vi "Read Firmware Version.vi"(8 "Error In":errorcluster, 11 "ChipKit Resource in":T1={"COM Port"="", "Board Type"=enum."ChipKit Uno32", "Connection Type"=enum."USB / Serial", "Baud Rate (115200)"=15, "Bytes Per Packet (15)"=15}) -> (0 "Error Out":errorcluster, 3 "ChipKit Resource out":T1={"COM Port"="", "Board Type"=enum."ChipKit Uno32", "Connection Type"=enum."USB / Serial", "Baud Rate (115200)"=15, "Bytes Per Packet (15)"=15})   [LabVIEW 2011, in "LabVIEW Interface for ChipKit.lvlib"]
uses:
  LabVIEW Interface for ChipKit.lvlib
  Private/Type Defs/Command.ctl
  Private/Type Defs/Board Type.ctl
  Private/Type Defs/Connection Type.ctl
  Private/Type Defs/Chipkit Resource.ctl
panel:
  out "Firmware Version":string
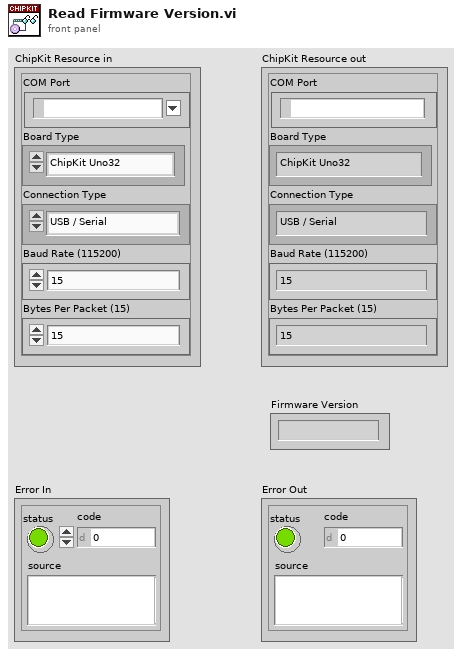
[diagram p1: front panel]
types:
  T1 = typedef "LabVIEW Interface for ChipKit.lvlib/Chipkit Resource.ctl" = cluster{"COM Port":refnum<visa-resource-name>, "Board Type":T2, "Connection Type":T3, "Baud Rate (115200)":u32, "Bytes Per Packet (15)":u32}
  T2 = typedef "LabVIEW Interface for ChipKit.lvlib/Board Type.ctl" = enum16{"ChipKit uC32", "ChipKit Uno32", "ChipKit Max32"}
  T3 = typedef "LabVIEW Interface for ChipKit.lvlib/Connection Type.ctl" = enum8{"USB / Serial", "XBEE", "BlueSmirf (Bluetooth)"}
  T4 = typedef "LabVIEW Interface for ChipKit.lvlib/Command.ctl" = enum8{"setArduinoMode", "flushSerial", "setPinMode", "digitalWritePin", "digitalWritePort", "tone", "digitalReadPin", "digitalReadPort", "analogReadPin", "analogReadPort", "pwmWritePin", "pwmWritePort", "sevenSegment_Configure", "sevenSegment_Write", "I2C Init", "I2C Write", "I2C Read", "SPI Init", "SPI Set Bit Order", "SPI Set Clock Divider", "SPI Set Data Mode", "SPI Send / Receive", "SPI Close", "Servo Set Num Servos", "Servo Config Servo", "Servo Write Angle", "Servo Read Angle", "Servo Write Pulse Width", "Servo Read Pulse Width", "Servo Detach", "LCD Init", "LCD Set Size", "LCD Set Cursor Mode", "LCD Clear", "LCD Set Cursor Position", "LCD Print", "LCD Display Power", "LCD Scroll Display", "LCD Autoscroll", "LCD Print Direction", "LCD Create Custom Char", "LCD Print Custom Char", "contAcqOn", "contAcqOff", "getFirmwareVersion", "FiniteSampleStart", "NA", "NA2", "Conifg Stepper", "Stepper Write", "Stepper Detach", "Stepper Steps To Go", "Config DO Port", "Config DI Port", "UART2 Open", "UART2 Write", "UART2 Bytes Available", "UART2 Read"}
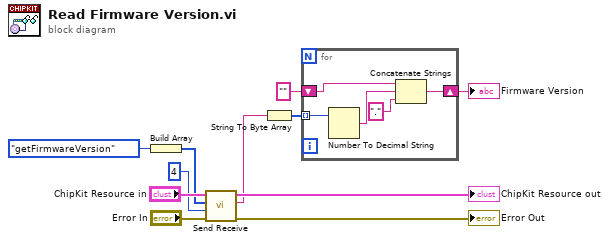
[diagram p0: block diagram]
diagram:
  n1 = Build Array(Command."getFirmwareVersion" ("Command")) -> (w6:T4[])
  n2 = call "Send Receive.vi"("Error In"="Error In", "Bytes To Read (0)"=u8 4, "Data"=w6, "ChipKit Resource"="ChipKit Resource in") -> ("Error Out"=→"Error Out":errorcluster, "Read Buffer"=w4:string, "ChipKit Resource"=→"ChipKit Resource out":T1)  [unwired: 5 in]
  n3 = String To Byte Array(string=w4) -> (unsigned byte array=w3:u8[])
  n4 = for {
    tunnel: w3 -> [w16] mode=indexing
    shift-right: [w13] -> w1
    shift-left: "" -> [w15]
    n5 = Number To Decimal String(number=w16) -> (decimal integer string=w14:string)  [unwired: 1 in]
    n6 = Concatenate Strings(w15, w14, "." ("string")) -> (w13:string)
  }
  "Firmware Version" <- w1
